vi "Avvia pompa.vi"(0 "Valvole avvio":T1, 1 "Tipo motore pompa":enum16{"Monofase", "Trifase"}(ring), 5 "Indici valvole linea":i16[](array[numeric]), 7 "V F rpm avvio":T2, 9 "V F rpm prova":T2, 12 "Reset avvio":bool) -> (6 "Fine Avvio":bool=TRUE, 10 "stato":string)   [LabVIEW 2019]
uses:
  Global_All_Data.vi
  cDAQ_PLC Folder/cDAQ/DO List.ctl
  cDAQ_PLC Folder/cDAQ/SET SINGLE DO.ctl
  cDAQ_PLC Folder/cDAQ/SET ARRAY DO.ctl
  cDAQ_PLC Folder/cDAQ/AO List.ctl
  cDAQ_PLC Folder/cDAQ/SET SINGLE AO.ctl
  SubVI ELETTROTEST60A Folder/Elettrotest60A/Global_bypass_ResMeter.vi
  Global SCELTA LINEA.vi
  Gestione Inverter/STATUS VACON.vi
panel:
  out "Stato":string
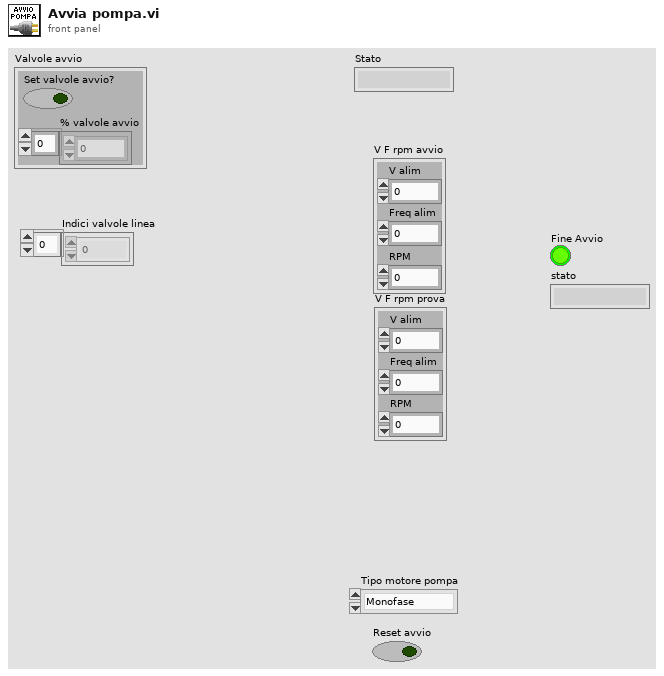
[diagram p1: front panel]
types:
  T1 = cluster{"Set valvole avvio?":bool, "% valvole avvio":dbl[]}
  T2 = cluster{"V alim":dbl, "Freq alim":dbl, "RPM":dbl}
  T3 = enum16{"Alimentazione diretta", "Variac/inverter", "Pompa trascinata"}
  T4 = enum16{"LINEA 135A BYPASS TRASFO", "LINEA 15A BYPASS TRASFO", "LINEA 135A TRASFO 400V", "LINEA 135A TRASFO 500V", "LINEA 15A TRASFO 400V", "LINEA 15A TRASFO 500V", "LINEA 2", "NESSUNA LINEA SELEZIONATA"}
  T5 = cluster{"Array of elements":cluster{"String":string, "variant":variant}[], "Single element":cluster{"String":string, "variant":variant}, "enque at\nopposite end (F)":bool, "no replications (F)":bool}
  T6 = typedef "SET ARRAY DO.ctl" = T7[]
  T7 = typedef "SET SINGLE DO.ctl" = cluster{"DO":T8, "Value":bool}
  T8 = typedef "DO List.ctl" = enum16{"OFF: ALL DO", "*ABILITA freno 1", "*ABILITA freno 2", "*ABILITA freno 3", "*START freno 1", "*START freno 2", "*START freno 3", "*STOP freno 1", "*STOP freno 3", "*STOP freno 2", "*Senso rot freno 1", "*Senso rot freno 2", "*Senso rot freno 3", "*Ctrl velocità freno 1", "*Ctrl velocità freno 2", "*Ctrl velocità freno 3", "*Ctrl coppia freno 1", "*Ctrl coppia freno 2", "*Ctrl coppia freno 3", "*ABILITA alimentatore 1", "*ABILITA alimentatore 2", "*ABILITA alimentatore 3", "*ABILITA alimentatore 4", "*START alimentatore 1", "*START alimentatore 2", "*START alimentatore 3", "*START alimentatore 4", "*STOP alimentatore 1", "*STOP alimentatore 2", "*STOP alimentatore 3", "*STOP alimentatore 4", "SENSO ROT alimentatore 1", "SENSO ROT alimentatore 2", "Abilita LEM 1000A", "Abilita LEM 300A", "Abilita sensori EXT WT", "B1 Seleziona linea 1", "B1 Seleziona linea 2", "B1 Seleziona linea 3", "B1 Seleziona linea 4", "B1 Seleziona linea 5", "B2 Seleziona linea 1", "B2 Seleziona linea 2", "B2 Seleziona linea 3", "B2 Seleziona linea 4", "B2 Seleziona linea 5", "*Reset allarmi", "*Start potenza AC", "*Stop potenza AC", "*Start potenza DC", "*Stop potenza DC", "*Start potenza DC eccit", "*Stop pontenza DC eccit", "Bypass res meter", "2nd canale res meter", "Enable res meter", "*Abilit teler ramo WT", "*Abil teler ramo princ Resit", "*Abil teler ramo 1 Resist", "*Abil teler ramo 2 Resist", "*Abil teler ramo 3 Resist", "*Abil cortocirc avvolgim", "*Controllo torsiometro B1", "*Controllo Torsiom B2", "*Scala torsiometro B1", "*Scala torsiometro B2", "*Collaudo in corso", "*Allarme presente", "Abilitazione elettroserratura", "Exit", "*Abilita collaudo", "*Abilita potenza trifase", "*Abilita potenza monofase", "*Abilita potenza DC", "*Abilita potenza DC eccit", "*Disabilita teleruttori potenza", "Set teleruttori prova a freddo", "Prova a freddo monofase", "Watchdog", "Forza DO PLC 3", "Forza DO PLC 2", "Forza DO PLC 1", "Forza DO cDAQ", "Scala 2000(T) 200(F) res meter", "Seleziona banco 1", "Seleziona banco 2", "Comando azionam in blocco", "Comando azionam reset", "Sensibilità freno 16 32 nm", "Reset Allarmi", "Carico res - Ramo 1", "Carico res - Ramo 2", "Carico res - Ramo 3", "Carico res - Ramo 4", "Carico res - Ramo 5", "Carico res - Ramo 6", "Carico res - Ramo 7", "Carico res - Ramo 8", "Carico res - Ramo 9", "Carico res - Ramo 10", "Carico res - Ramo 11", "Carico res - Start ventilatore", "Carico res - Stop ventilatore", "Abilita potenza solo freno", "Abilita AFE + freno trasc", "Abilita potenza carico resistivo", "Chiudi potenza AFE", "Apri potenza AFE", "Start AFE", "Config Banco2 TDE", "Misura diretto WT", "Ripristina centralina protezioni", "Abilita Scrittura Dati Keb"}
  T9 = typedef "SET SINGLE AO.ctl" = cluster{"AO":T10, "Value":dbl}
  T10 = typedef "AO List.ctl" = enum16{"OFF: ALL AO", "Valvola prop 1", "Valvola prop 2", "Valvola prop 3", "Valvola prop 4", "Valvola prop 5", "Valvola prop 6", "Vavlola prop 7", "Valvola prop 8", "Valvola prop 9", "Valvola prop 10", "Rif vel motore trasc 1", "Rif vel motore trasc 2", "Rif vel motore trasc 3", "Rif vel motore pompa boost 1", "Rif vel motore pompa boost 2", "Rif vel motore pompa boost 3", "Rif Vout", "Rif Freq out", "FORZA AO", "Exit"}
  T11 = typedef "Cluster MISURE.ctl" = cluster{"MISURE NM":T12, "MISURE ALL":T13}
  T12 = typedef "MISURE NM.ctl" = cluster{"Banco":string, "Anno":string, "Numero":string, "Ntabella":string, "Misura":string, "Tipo Prova":string, "ProgressivoAcq":string, "Descrizione":string, "Data_ora":string, "t. acq [h:m:s]":string, "t. acq [min]":string, "t. acq [s]":string, "n [rpm]":string, "f [Hz]":string, "U1[V]":string, "U2 [V]":string, "U3 [V]":string, "U123_media [V]":string, "I1[A]":string, "I2[A]":string, "I3[A]":string, "I123_media [A]*I":string, "I_123_sbil [%]":string, "Ulin[V]":string, "Uc [V]":string, "Uaux [V]":string, "Ilin[A]*I":string, "Imar[A]":string, "Iaux[A]":string, "Uarm[V]":string, "Uecc[V]":string, "Iarm[A]*I":string, "Iecc[A]":string, "pf":string, "P1 [W]":string, "P1 [kW]":string, "Q [VAR]":string, "Q [kVAR]":string, "S [VA]":string, "S [kVA]":string, "P1arm[W]":string, "P1ecc[W]":string, "Parm[kW]":string, "P1ecc[kW]":string, "Cond[uF]":string, "P1_linea_6fili[W]":string, "P1_linea_6fili[kW]":string, "eta_gr_6fili [%]":string, "eta_inverter_6fili [%]":string, "pf_linea_6fili":string, "U4 [V]":string, "U5 [V]":string, "U6 [V]":string, "U456_media [V]":string, "I4 [A]":string, "I5 [A]":string, "I6 [A]":string, "I456_media [A]":string, "C [Nm]*C":string, "Cric [Nm]":string, "Cric\\Cnom":string, "Iric[A]":string, "Iric\\Inom":string, "P2_mecc [W]":string, "P2_mecc [kW]":string, "eta motore [%]":string, "Scorr[%]":string, "Tamb[°C]":string, "R1[ohm]":string, "R2[ohm]":string, "R3[ohm]":string, "Rmedia[ohm]":string, "DT_R1[°C]":string, "DT_R2[°C]":string, "DT_R3[°C]":string, "DT_media[°C]":string, "R_marcia[ohm]":string, "R_aux[ohm]":string, "DT_marcia[°C]":string, "DT_aux[°C]":string, "R_Arm[ohm]":string, "R_Ecc[ohm]":string, "DT_Arm[°C]":string, "DT_Ecc[°C]":string, "TambFreddo[°C]":string, "R1_freddo[ohm]":string, "R2_freddo[ohm]":string, "R3_freddo[ohm]":string, "Rmedia_freddo[ohm]":string, "R_Marcia_freddo[ohm]":string, "R_Aux_freddo[ohm]":string, "R_Arm_freddo[ohm]":string, "R_Ecc_freddo[ohm]":string, "TC1 [°C]":string, "TC2 [°C]":string, "TC3 [°C]":string, "TC4 [°C]":string, "TC5 [°C]":string, "TC6 [°C]":string, "TC7 [°C]":string, "TC8 [°C]":string, "PT1000_1[°C]":string, "PT1000_2[°C]":string, "PT1000_3[°C]":string, "Vdc eccitatrice[V]":string, "Idc eccitatrice[A]":string, "Vdc rotore[V]":string, "Idc rotore[A]":string, "Vac rotore[V]":string, "Iac rotore[V]":string, "V dinamo[V]":string, "Portata Q":string, "Pressione H":string, "U1'[V]":string, "U2'[V]":string, "U3'[V]":string, "I1'[A]":string, "I2'[A]":string, "I3'[A]":string, "U''R-N":string, "U''S-N":string, "U'' T-N":string, "U''R-S":string, "U''R-T":string, "U''S-T":string, "I1''[A]":string, "I2''[A]":string, "I3''[A]":string, "F''[Hz]":string, "P''[kW]":string, "CosFi''":string, "PT1000_4[°C]":string, "Scorta 3":string}
  T13 = typedef "Cluster misure ALL.ctl" = cluster{"Cluster READ NI":T14, "MISURE WT":T17, "Resistenze Resistomat":T18, "INTERFACCIA":T19, "FREDDO resistomat":cluster{"Res Ch1":dbl, "Res Ch2":dbl, "tAMB":dbl, "Res Ch3":dbl}, "STATO PLC 1":T24, "Res Ch2":dbl, "Res Ch2 2":dbl, "FREDDO res meter":cluster{"Res Ch1":dbl, "Res Ch2":dbl, "tAMB":dbl, "Res Ch3":dbl}, "Resistenze Res Meter":T18, "READ SINUS PENTA":T28, "STATO PLC 2":T29, "STATO PLC 3":T33, "DCREG":T37}
  T14 = typedef "Cluster NI.ctl" = cluster{"AI (0-10V)":cluster{"AI 0":dbl, "AI 1":dbl, "AI 2":dbl, "AI 3":dbl, "AI 4":dbl, "AI 5":dbl, "AI 6":dbl, "AI 7":dbl, "AI 8":dbl, "AI 9":dbl, "AI 10":dbl, "AI 11":dbl, "AI 12":dbl, "AI 13":dbl, "AI 14":dbl, "AI 15":dbl, "AI 16":dbl, "AI 17":dbl, "AI 18":dbl, "AI 19":dbl, "AI 20":dbl, "AI 21":dbl, "AI 22":dbl, "AI 23":dbl, "AI 24":dbl, "AI 25":dbl, "AI 26":dbl, "AI 27":dbl, "AI 28":dbl, "AI 29":dbl, "AI 30":dbl, "AI 31":dbl}, "StatoAO_Cdaq[0-10V]":cluster{"AO 1":dbl, "AO 2":dbl, "AO 3":dbl, "AO 4":dbl}, "Contatori [rpm]":cluster{"RPM 1":dbl, "RPM 2":dbl}, "StatoAO_Cdaq [4-20mA]":T15, "StatoDO_Cdaq":T16, "DI":cluster{"Scorta 0":bool, "Scorta 1":bool, "Scorta 2":bool, "Scorta 3":bool, "Scorta 4":bool, "Scorta 5":bool, "Scorta 6":bool, "Scorta 7":bool, "Scorta 8":bool, "Scorta 9":bool, "Scorta 10":bool, "Scorta 11":bool, "Scorta 12":bool, "Scorta 13":bool, "Scorta 14":bool, "Scorta 15":bool, "Scorta 16":bool, "Scorta 17":bool, "Scorta 18":bool, "Scorta 19":bool, "Scorta 20":bool, "Scorta 21":bool, "Scorta 22":bool, "Scorta 23":bool, "Scorta 24":bool, "Scorta 25":bool, "Scorta 26":bool, "Scorta 27":bool, "Scorta 28":bool, "Scorta 29":bool, "Scorta 30":bool, "Scorta 31":bool}, "AI (4-20mA)":cluster{"AI 0":dbl, "AI 1":dbl, "AI 2":dbl, "AI 3":dbl, "AI 4":dbl, "AI 5":dbl, "AI 6":dbl, "AI 7":dbl, "AI 8":dbl, "AI 9":dbl, "AI 10":dbl, "AI 11":dbl, "AI 12":dbl, "AI 13":dbl, "AI 14":dbl, "AI 15":dbl}, "TC [°C]":cluster{"tc 1":dbl, "tc 2":dbl, "tc 3":dbl, "tc 4":dbl}}
  T15 = typedef "StatoAO_cdaq.ctl" = cluster{"Cdaq_AO [0-10V] 0":dbl, "Cdaq_AO [0-10V] 1":dbl, "Cdaq_AO [0-10V] 2":dbl, "Cdaq_AO [0-10V] 3":dbl, "Cdaq_AO [4-20mA] 0":dbl, "Cdaq_AO [4-20mA] 1":dbl, "Cdaq_AO [4-20mA] 2":dbl, "Cdaq_AO [4-20mA] 3":dbl, "Cdaq_AO [4-20mA] 4":dbl, "Cdaq_AO [4-20mA] 5":dbl, "Cdaq_AO [4-20mA] 6":dbl, "Cdaq_AO [4-20mA] 7":dbl}
  T16 = typedef "statoDO_Cdaq.ctl" = cluster{"Scorta 0":bool, "Scorta 1":bool, "Scorta 2":bool, "Scorta 3":bool, "Scorta 4":bool, "Scorta 5":bool, "Scorta 6":bool, "Scorta 7":bool, "Scorta 8":bool, "Scorta 9":bool, "Scorta 10":bool, "Scorta 11":bool, "Scorta 12":bool, "Scorta 13":bool, "Scorta 14":bool, "Scorta 15":bool, "Scorta 16":bool, "Scorta 17":bool, "Scorta 18":bool, "Scorta 19":bool, "Scorta 20":bool, "Scorta 21":bool, "Scorta 22":bool, "Scorta 23":bool, "Scorta 24":bool, "Scorta 25":bool, "Scorta 26":bool, "Scorta 27":bool, "Scorta 28":bool, "Scorta 29":bool, "Scorta 30":bool, "Scorta 31":bool}
  T17 = typedef "MISURE WT.ctl" = cluster{"URMS 1":dbl, "IRMS 1":dbl, "P 1":dbl, "S 1":dbl, "Q 1":dbl, "LAMBDA 1":dbl, "PHI 1":dbl, "F U 1":dbl, "F I 1":dbl, "NONE 1":dbl, "URMS 2":dbl, "IRMS 2":dbl, "P 2":dbl, "S 2":dbl, "Q 2":dbl, "LAMBDA 2":dbl, "PHI 2":dbl, "F U 2":dbl, "F I 2":dbl, "NONE 2":dbl, "URMS 3":dbl, "IRMS 3":dbl, "P 3":dbl, "S 3":dbl, "Q 3":dbl, "LAMBDA 3":dbl, "PHI 3":dbl, "F U 3":dbl, "F I 3":dbl, "NONE 3":dbl, "URMS 4":dbl, "IRMS 4":dbl, "P 4":dbl, "S 4":dbl, "Q 4":dbl, "LAMBDA 4":dbl, "PHI 4":dbl, "F U 4":dbl, "F I 4":dbl, "NONE 4":dbl, "URMS 5":dbl, "IRMS 5":dbl, "P 5":dbl, "S 5":dbl, "Q 5":dbl, "LAMBDA 5":dbl, "PHI 5":dbl, "F U 5":dbl, "F I 5":dbl, "NONE 5":dbl, "URMS 6":dbl, "IRMS 6":dbl, "P 6":dbl, "S 6":dbl, "Q 6":dbl, "LAMBDA 6":dbl, "PHI 6":dbl, "F U 6":dbl, "F I 6":dbl, "NONE 6":dbl, "URMS SIGMA":dbl, "IRMS SIGMA":dbl, "P SIGMA":dbl, "S SIGMA":dbl, "Q SIGMA":dbl, "LAMBDA SIGMA":dbl, "PHI SIGMA":dbl, "F U SIGMA":dbl, "F I SIGMA":dbl, "NONE 7":dbl, "URMS SIGMB":dbl, "IRMS SIGMB":dbl, "P SIGMB":dbl, "S SIGMB":dbl, "Q SIGMB":dbl, "LAMBDA SIGMB":dbl, "PHI SIGMB":dbl, "F U SIGMB":dbl, "F I SIGMB":dbl, "NONE 8":dbl, "URMS SIGMC":dbl, "IRMS SIGMC":dbl, "P SIGMC":dbl, "S SIGMC":dbl, "Q SIGMC":dbl, "LAMBDA SIGMC":dbl, "PHI SIGMC":dbl, "F U SIGMC":dbl, "F I SIGMC":dbl, "NONE 9":dbl, "SPEED":dbl, "TORQUE[Nm]":dbl, "Pmecc[kW]":dbl}
  T18 = typedef "ClusterRes.ctl" = cluster{"Res Ch1":dbl, "Res Ch2":dbl, "Res Ch3":dbl, "Tamb":dbl}
  T19 = typedef "INTERFACCIA.ctl" = cluster{"AI":cluster{"Portate":T20[], "Pressioni":T20[], "Coppie[Nm]":T20[], "Valvole prop %":T20[], "RPM":T20[], "Livelli":T20[], "Temperature":T20[], "Riferimenti %":T20[], "TENSIONI":T20[], "CORRENTI":T20[]}, "DI (logici)":cluster{"Start da pulsantiera":bool, "Stop da pulsantiera":bool, "Reset da pulsantiera":bool, "Sistema OK":bool, "Collaudo abilitato":bool, "Potenza trifase abilitata":bool, "Potenza monofase abilitata":bool, "Potenza DC abilitata":bool, "Potenza DC ECC abilitata":bool, "Start alimentazione AC":bool, "Start alimentazione DC":bool, "Start DC eccitazione":bool, "Teleruttore WT abilitato":bool, "Teleruttore Resistomat abilitato":bool, "Teleruttore corto fasi":bool, "Ramo 1 resistomat":bool, "Ramo 2 resistomat":bool, "Ramo 3 resistomat":bool, "B1 Scelta linea elettrica 1":bool, "B1 Scelta linea elettrica 2":bool, "B1 Scelta linea elettrica 3":bool, "B1 Scelta linea elettrica 4":bool, "B1 Scelta linea elettrica 5":bool, "B2 Scelta linea elettrica 1":bool, "B2 Scelta linea elettrica 2":bool, "B2 Scelta linea elettrica 3":bool, "B2 Scelta linea elettrica 4":bool, "B2 Scelta linea elettrica 5":bool, "Rotore bloccato 1":bool, "Rotore bloccato 2":bool, "FRENO 1 abilitato":bool, "FRENO 1 run":bool, "FRENO 1 senso rotaz":bool, "FRENO 1 ctrl velocità":bool, "FRENO 2 abilitato":bool, "FRENO 2 run":bool, "FRENO 2 senso rotaz":bool, "FRENO 2 ctrl velocità":bool, "ALIM 1 abilitato":bool, "ALIM 1 run":bool, "ALIM 2 abilitato":bool, "ALIM 2 run":bool, "ALIM 3 abilitato":bool, "ALIM 3 run":bool, "FRENO 1 ctrl coppia":bool, "FRENO 2 ctrl coppia":bool, "FRENO 3 ctrl coppia":bool, "DI (logici) aggiuntivi impianto":cluster{"Solo freno abilitato":bool, "Carico resistivo abilitato":bool, "AFE+freno abilitato":bool, "Protezioni chiuse":bool, "Start potenza AFE":bool, "AFE in marcia":bool}, "Misura corrente diretta WT":bool, "Misura corrente sens ext":bool, "Sens ext abilitati":bool}, "AO non scalati":T22, "AO scalati":T22, "DO (logici)":T23}
  T20 = typedef "ClusterMisura_e_Unità_INPUT.ctl" = cluster{"Misura":dbl, "UM":T21, "Descrizione":string}
  T21 = typedef "UnitàMisura.ctl" = enum16{"V", "mA", "Bar", "RPM", "m3/s", "m3/min", "m3/h", "l/s", "l/min", "in3/min", "ft3/min", "gpm", "igpm", "igph", "%", "°C", "m", "Nm", "A"}
  T22 = typedef "Lista AO sistema.ctl" = cluster{"FRENO1 rif vel":dbl, "FRENO1 rif Coppia":dbl, "FRENO2 rif vel":dbl, "FRENO2 rif Coppia":dbl, "ALIM1 rif V":dbl, "ALIM1 rif F":dbl, "ALIM2 rif V":dbl, "ALIM2 rif F":dbl, "ALIM3 rif V":dbl, "ALIM3 rif F":dbl, "Fnom keb":dbl, "Rpm nom keb":dbl, "Pnom keb":dbl, "Inom keb":dbl, "Vnom keb":dbl, "Rpm max keb":dbl, "Tempo rampa keb":dbl, "Tipo Mot keb":dbl}
  T23 = typedef "DOinterfaccia.ctl" = cluster{"Scelta banco 1":bool, "Scelta banco 2":bool, "Scelta banco 3":bool, "FRENO 1 abilita":bool, "FRENO 1 start":bool, "FRENO 1 senso rotaz":bool, "FRENO 1 ctrl velocità":bool, "FRENO 2 abilita":bool, "FRENO 2 start":bool, "FRENO 2 senso rotaz":bool, "FRENO 2 ctrl velocità":bool, "ALIM 1 abilita":bool, "ALIM 1 start":bool, "ALIM 2 abilita":bool, "ALIM 2 start":bool, "ALIM 3 abilita":bool, "ALIM 3 start":bool, "Abilita linea trifase":bool, "Abilita linea monofase":bool, "Abilita linea dc":bool, "Abilita linea dc eccit":bool, "B1 Linea elettrica 1":bool, "B1 Linea elettrica 2":bool, "B1 Linea elettrica 3":bool, "B1 Linea elettrica 4":bool, "B1 Linea elettrica 5":bool, "B2 Linea elettrica 1":bool, "B2 Linea elettrica 2":bool, "B2 Linea elettrica 3":bool, "B2 Linea elettrica 4":bool, "B2 Linea elettrica 5":bool, "Start potenza AC":bool, "Stop pontenza AC":bool, "Start potenza DC":bool, "Stop potenza DC":bool, "Start potenza eccitaz":bool, "Stop potenza eccitaz":bool, "Reset allarmi":bool, "watchdog":bool, "Scala torsiometro B1":bool, "Controllo torsiom B1":bool, "Scala torsiometro B2":bool, "Controllo torsiom B2":bool, "Teleruttore WT abilita":bool, "Teleruttore Resistomat abilita":bool, "Teleruttore corto fasi":bool, "Ramo 1 resistomat":bool, "Ramo 2 resistomat":bool, "Ramo 3 resistomat":bool, "Collaudo in corso":bool, "Allarme presente":bool, "Enable Res Meter":bool, "Bypass Res Meter":bool, "2nd canale Res Meter":bool, "Scala 200/2000 res meter":bool, "Taratura res meter":bool, "FRENO 1 ctrl coppia":bool, "FRENO 2 ctrl coppia":bool, "FRENO 3 ctrl coppia":bool, "Aggiuntivi impianto":cluster{"Senso rotazione alim 1":bool, "Senso rotazione alim 2":bool}, "ALIM 1 stop":bool, "ALIM 2 stop":bool, "ALIM 3 stop":bool, "FRENO 1 stop":bool, "FRENO 2 stop":bool, "FRENO 3 stop":bool, "B1 configurazione freno B":bool, "B2 configurazione freno B":bool, "Abilita scrittura KEB":bool}
  T24 = typedef "STATO PLC 1.ctl" = cluster{"USCITE PLC":T25, "Stato DI_PLC":cluster{"Sistema OK":bool, "Rotore bloccato":bool, "Scorta 1":bool, "Prova diretto inverter":bool, "Prova con filtro LC":bool, "Teleruttore WT abilitato":bool, "Alim sinus penta abilitato":bool, "Alim sinus penta in marcia":bool, "Freno abilitato":bool, "Freno in marcia":bool, "Senso rotazione freno":bool, "Potenza abilitata":bool, "Scorta 3":bool, "Scorta 4":bool, "scorta 5":bool, "scorta 6":bool}, "AI plc":cluster{"Allarmi 1":dbl, "Allarmi 2":dbl, "Scorta 1":dbl, "Scorta 2":dbl, "RPM mot prova":dbl, "I mot prova":dbl, "RPM freno":dbl, "I freno":dbl, "Scorta 3":dbl, "Scorta 4":dbl}}
  T25 = typedef "Uscite PLC 1.ctl" = cluster{"AO (real) 2":cluster{"SCORTA 1":dbl, "SCORTA 2":dbl, "SCORTA 3":dbl, "SCORTA 4":dbl, "SCORTA 5":dbl, "SCORTA 6":dbl, "SCORTA 7":dbl, "SCORTA 8":dbl}, "statoAO_PLC out":T26, "DO (bit)":T27}
  T26 = typedef "statoAO_plc_1.ctl" = cluster{"Rif Lim coppia freno [%]":dbl, "Rif rpm freno [%]":dbl, "Rif coppia freno [%]":dbl, "Rif V alimentatore [%]":dbl, "Rif F alimentatore [%]":dbl}
  T27 = typedef "StatoDO_PLC_1.ctl" = cluster{"Scelta banco 1":bool, "Set dati motore freno 2":bool, "Diretto inverter":bool, "Filtro LC":bool, "Marcia ALIM (1s)":bool, "Marcia FRENO (1s)":bool, "Stop AFE (1s)":bool, "Stop freno (1s)":bool, "Reset allarmi":bool, "Watchdog":bool, "Senso rotazione":bool, "Abilita collaudo (1s)":bool, "Disabilita collaudo (1s)":bool, "Abilitazione ALIM":bool, "Abilitazione FRENO":bool, "Teleruttore WT":bool, "Senso rot motore prova":bool, "Scorta 7":bool, "Scorta 8":bool, "Scorta 9":bool, "Scorta 10":bool, "Scorta 11":bool, "Scorta 12":bool, "Scorta 13":bool}
  T28 = typedef "Parametri inverter letti.ctl" = cluster{"Menù Misure motore (M000-M030)":cluster{"Rif vel a regime (int)":u16, "Rif vel a regime (dec)":u16, "Rif vel dopo rampe (int)":u16, "Rif vel dopo rampe (dec)":u16, "RPM motore (int)":u16, "RPM motore (dec)":u16, "FREQout inverter":u16, "Rif coppia a regime(Nm)":u16, "Richiesta di coppia (Nm)":u16, "Coppia generata dal motore(Nm)":u16, "Rif coppia a regime(%)":u16, "Richiesta di coppia (%)":u16, "Coppia generata dal motore(%)":u16, "Coppia max richiesta prima delle rampe(Nm)":u16, "Coppia max richiesta dopo le rampe(Nm)":u16, "Limite di velocità prima delle rampe":u16, "Limite di velocità dopo le rampe":u16, "Coppia max richiesta prima delle rampe(%)":u16, "Coppia max richiesta dopo le rampe(%)":u16, "Rif di flusso":u16, "Corrente di uscita":u16, "Capacità termica del motore":u16, "Tensione di uscita":u16, "Potenza di uscita":u16, "Energia consumata (LSword)":u16, "Energia consumata (MSword)":u16, "Tensione bus DC":u16, "Tensione di rete":u16}, "Menù regolatore PID (M018-M024)":cluster{"Rif PID a regime(%)":u16, "Rif pid dopo rampe(%)":u16, "Retroazione del pid(%)":u16, "Errore del pid(%)":u16, "uscita del pid(%)":u16, "Rif del pid dopo le rampe":u16, "Retroazione del pid":u16}, "Menù ingressi digitali (M031-M036)":cluster{"Ingressi digitali ritardati":u16, "Ingressi digitali istantanei":u16, "Moresettiera comando loc":u16, "Morsett comando da seriale":u16, "Morsett comando bus di campo":u16, "Ing dig ausiliari da morsettiera":u16, "Ing dig ausiliari da seriale":u16}, "Menù riferimenti (M037-M051)":cluster{"Rif analog est REF":u16, "Rif analog est AIN1":u16, "Rif analog est AIN2":u16, "Rif analog est XAIN4":u16, "Rif analog est XAIN5":u16, "Rif velocità da seriale(int)":u16, "Rif velocità bus di campo(int)":u16, "Rif coppia da seriale":u16, "Rif coppia bus di campo":u16, "Rif del PID da seriale":u16, "Rif del PID da bus di campo":u16, "Retroazione del PID da seriale":u16, "Retroazione del PIDda bus di campo":u16, "Rif da encoder":u16, "Rif in frequenza":u16, "Rif velocità da seriale(dec)":u16, "Rif velocità bus di campo(dec)":u16}, "Menù rampe (P009-P033)":cluster{"Tempo di dec rampa di vel 1":u16, "Tempo di acc rampa di vel 2":u16, "Tempo di dec rampa di vel 2":u16, "Tempo di acc rampa di vel 1":u16, "Unità di mis tempi rampe vel 1/2":u16, "Tempo di acc rampa di vel 3":u16, "Tempo di dec rampa di vel 3":u16, "Tempo di acc rampa di vel 4":u16, "Tempo di dec rampa di vel 4":u16, "Unità di mis tempi rampe vel 3/4":u16, "Selettore arrottondam rampe":u16, "Tempo di arrotond iniz rampa acc":u16, "Tempo di arrotond finale rampa acc":u16, "Tempo di arrotond iniz rampa dec":u16, "Tempo di rampa di salita rif coppia":u16, "Tempo di rampa di discesa rif coppia":u16, "Unità di misura rampa coppia":u16, "Tempo rampa acc marcia jog":u16, "Tempo rampa dec marcia jog":u16, "Reset acc ai cambi pendenza":u16, "rampa di acc in fire mode":u16, "rampa di dec in fire mode":u16, "Tempo di arrotond finale rampa dec":u16}, "Menù controllo motore(C008-C128)":cluster{"Numero motori configurati":u16, "Tipo algoritmo di controllo Mot1":u16, "Tipo rif Mot1":u16, "Tensione nominale rete":u16, "Retroaz di vel da encoder Mot1":u16, "Tipo curva V/f Mot1":u16, "Rotazione delle fasi Mot1":u16, "Freq nominale del motore Mot1":u16, "RPM nominali del motore Mot1":u16, "Potenza nominale del motore Mot1":u16, "Corrente nominale del motore Mot1":u16, "Tensione nominale del motore mot1":u16, "Potenza a vuoto del motore Mot1":u16, "Corrente a vuoto del motore Mot1":u16, "Resistenza statorica del motore Mot1":u16, "Induttanza di dispersione Mot1":u16, "Induttanza mutua motore":u16, "Costante di tempo rotorica":u16, "Costante di tempo filtro pb":u16, "Velocità minima motore":u16, "Velocità massima motore":u16}, "Menù configurazione PID":cluster{"Selezione riferimento n.1":u16, "Selezione retroazione n.1":u16, "Modalità di fuzionamento PID":u16, "Termine derivativo calcolato su err o mis":u16, "Proporz moltiplica deriv e integrale":u16, "Azione del PID":u16}, "ID":dbl, "Menù uscite digitali":cluster{"MDO4 Inverter pronto":u16}, "Fcarrier":cluster{"Fcarrier Min (Hz)":u16, "Fcarrier Max (Hz)":u16}, "stato inverter M089":dbl, "Riferimenti":cluster{"Rif tensione":u16, "Rif velocità":u16}, "Comunicazione":bool, "Modalità stop":dbl}
  T29 = typedef "STATO PLC 2.ctl" = cluster{"USCITE PLC":T30, "Stato DI_PLC":cluster{"Sistema ok":bool, "Relè Resistomat abilitato":bool, "scorta d":bool, "scorta c":bool, "scorta b":bool, "scorta a":bool, "scorta 1":bool, "scorta 2":bool, "scorta 3":bool, "scorta 4":bool, "Scorta 5":bool, "Scorta 6":bool, "Scorta 7":bool, "Scorta 8":bool, "Scorta 9":bool, "Scorta 10":bool}, "AI plc":cluster{"Allarmi 1":dbl, "Allarmi 2":dbl, "TC 1":dbl, "TC 2":dbl, "TC 3":dbl, "TC 4":dbl, "TC 5":dbl, "TC 6":dbl, "TC 7":dbl, "TC 8":dbl, "PT1000 1":dbl, "PT1000 2":dbl, "PT1000 3":dbl, "PT1000 4":dbl}}
  T30 = typedef "Uscite PLC 2.ctl" = cluster{"AO (real) 2":cluster{"SCORTA 1":dbl, "SCORTA 2":dbl, "SCORTA 3":dbl, "SCORTA 4":dbl, "SCORTA 5":dbl, "SCORTA 6":dbl, "SCORTA 7":dbl, "SCORTA 8":dbl}, "statoAO_PLC out":T31, "DO (bit)":T32}
  T31 = typedef "statoAO_plc_2.ctl" = cluster{"Condensatori":dbl, "Scorta 1":dbl, "Scorta 2":dbl}
  T32 = typedef "StatoDO_PLC_2.ctl" = cluster{"Scala Torsiometro":bool, "Ctrl torsiometro":bool, "Relè misura resistomat":bool, "Watchdog":bool, "Misura res ramo 1":bool, "Misura res ramo 2":bool, "Misura res ramo 3":bool, "Scelta banco 2":bool, "Reset allarmi":bool, "Reset centraline":bool, "Scorta 2":bool, "Scorta 3":bool, "Scorta 4":bool, "Scorta 5":bool, "Scorta 6":bool, "Scorta 7":bool}
  T33 = typedef "STATO PLC 3.ctl" = cluster{"USCITE PLC":T34, "Stato DI_PLC":cluster{"Sistema OK":bool, "Rotore bloccato":bool, "Filtro LC":bool, "Bypass Filtro LC":bool, "Scelta Trasformatore":bool, "Scelta Bypass trasformatore":bool, "Teleruttore wt abilitato":bool, "Alimentatore abilitato":bool, "Alimentatore in marcia":bool, "Freno abilitato":bool, "Freno in marcia":bool, "Freno senso di rotazione":bool, "Potenza abilitata":bool, "Alimentatore in allarme":bool, "Freno in allarme":bool, "Conferma dati KEB":bool, "Scorta 4":bool, "Scorta 5":bool, "Scorta 6":bool}, "AI plc":cluster{"Allarmi 1":dbl, "Allarmi 2":dbl, "RPM motore prova":dbl, "Corrente motore prova":dbl, "RPM freno":dbl, "Corrente freno":dbl, "Tipo motore keb":dbl, "I nom keb":dbl, "RPM nom keb":dbl, "V nom keb":dbl, "F nom keb":dbl, "T rampa keb":dbl, "scorta":dbl, "Scorta 2":dbl}}
  T34 = typedef "Uscite PLC 3.ctl" = cluster{"AO (real) 2":cluster{"SCORTA 1":dbl, "SCORTA 2":dbl, "SCORTA 3":dbl, "SCORTA 4":dbl, "SCORTA 5":dbl, "SCORTA 6":dbl, "SCORTA 7":dbl, "SCORTA 8":dbl}, "statoAO_PLC out":T35, "DO (bit)":T36}
  T35 = typedef "statoAO_plc_3.ctl" = cluster{"Rif limitazione coppia freno":dbl, "Rif velocità freno":dbl, "Rif coppia freno (predisp.)":dbl, "Rif velocità alimentatore":dbl, "Scorta":dbl, "Tipo Motore  keb":dbl, "I nom keb":dbl, "RPM nom keb":dbl, "V nom keb":dbl, "F nom keb":dbl, "t rampa keb":dbl, "scorta":dbl, "Scorta 2":dbl}
  T36 = typedef "StatoDO_PLC_3.ctl" = cluster{"Scelta banco 2":bool, "Abilita Scrittura Dati Keb":bool, "Filtro LC":bool, "Bypass filtro LC":bool, "Trasformatore":bool, "Bypass trasformatore":bool, "Marcia alimentatore (1s)":bool, "Marcia freno (1s)":bool, "Stop alimentatore (1s)":bool, "Stop freno (1s)":bool, "Reset allarmi":bool, "Watchdog":bool, "Freno senso di rotazione":bool, "Abilita pontenza (1s)":bool, "Disabilita potenza (1s)":bool, "Abilita alimentatore":bool, "Abilita freno":bool, "Teleruttore wt":bool, "Senso rot mot prova":bool, "Scorta":bool, "Scorta":bool, "Blocco elettroserrature":bool, "Scorta 6":bool, "Scorta 7":bool}
  T37 = typedef "Parametri DCREG letti.ctl" = cluster{"Parametri di misura":cluster{"M000":dbl, "M001":dbl, "M002":dbl, "M003":dbl, "M004":dbl, "M005":dbl, "M006":dbl, "M007":dbl, "M008":dbl, "M009":dbl, "M010":dbl, "M011":dbl, "M012":dbl, "M013":dbl, "M014":dbl, "M015":dbl, "M016":dbl, "M017":dbl, "M018":dbl, "M019":dbl, "M020":dbl, "M021":dbl, "M022":dbl, "M023":dbl, "M024":dbl, "M025":dbl, "M026":dbl, "M027":dbl, "M028":dbl, "M029":dbl, "M030":dbl, "M031":dbl}, "Parametri di programmazione":cluster{"P000":dbl, "P001":dbl, "P002":dbl, "P003":dbl, "P004":dbl, "P005":dbl, "P006":dbl, "P010":dbl, "P011":dbl, "P012":dbl, "P013":dbl, "P014":dbl, "P015":dbl, "P016":dbl, "P030":dbl, "P031":dbl, "P032":dbl, "P033":dbl, "P034":dbl, "P035":dbl, "P036":dbl, "P037":dbl, "P038":dbl, "P039":dbl, "P040":dbl, "P050":dbl, "P051":dbl, "P052":dbl, "P053":dbl, "P054":dbl, "P055":dbl, "P056":dbl, "P057":dbl, "P058":dbl, "P059":dbl, "P060":dbl, "P061":dbl, "P062":dbl, "P070":dbl, "P071":dbl, "P073":dbl, "P074":dbl, "P076":dbl, "P077":dbl, "P079":dbl, "P080":dbl, "P082":dbl, "P083":dbl, "P084":dbl, "P085":dbl, "P086":dbl, "P087":dbl, "P088":dbl, "P100":dbl, "P101":dbl, "P102":dbl, "P103":dbl, "P104":dbl, "P110":dbl, "P111":dbl, "P120":dbl, "P121":dbl, "P122":dbl, "P123":dbl, "P124":dbl, "P125":dbl, "P126":dbl, "P127":dbl, "P128":dbl, "P129":dbl, "P130":dbl, "P131":dbl, "P132":dbl, "P133":dbl, "P134":dbl, "P150":dbl, "P151":dbl, "P152":dbl, "P153":dbl, "P154":dbl, "P155":dbl, "P156":dbl, "P157":dbl, "P158":dbl, "P170":dbl, "P171":dbl, "P172":dbl, "P173":dbl, "P174":dbl, "P175":dbl, "P176":dbl, "P177":dbl, "P178":dbl, "P179":dbl, "P180":dbl, "P181":dbl, "P182":dbl, "P183":dbl, "P184":dbl, "P185":dbl, "P186":dbl, "P187":dbl, "P188":dbl, "P189":dbl, "P190":dbl, "P191":dbl, "P192":dbl, "P193":dbl, "P194":dbl, "P195":dbl, "P196":dbl, "P197":dbl, "P198":dbl, "P199":dbl, "P211":dbl, "P212":dbl, "P213":dbl, "P214":dbl, "P215":dbl, "P216":dbl, "P217":dbl, "P221":dbl, "P222":dbl, "P223":dbl, "P224":dbl, "P230":dbl, "P231":dbl, "P240":dbl, "P250":dbl, "P251":dbl}, "Parametri di configurazione":cluster{"C000":dbl, "C001":dbl, "C002":dbl, "C010":dbl, "C011":dbl, "C012":dbl, "C014":dbl, "C015":dbl, "C016":dbl, "C017":dbl, "C018":dbl, "C030":dbl, "C050":dbl, "C051":dbl, "C052":dbl, "C060":dbl, "C061":dbl, "C062":dbl, "C063":dbl, "C070":dbl, "C072":dbl, "C074":dbl, "C090":dbl, "C091":dbl, "C092":dbl, "C093":dbl, "C094":dbl, "C100":dbl, "C101":dbl, "C102":dbl, "C103":dbl, "C105":dbl, "C106":dbl, "C107":dbl, "C108":dbl, "C110":dbl, "C111":dbl, "C112":dbl, "C120":dbl, "C121":dbl, "C122":dbl, "C130":dbl, "C131":dbl, "C132":dbl, "C133":dbl, "C134":dbl, "C135":dbl, "C141":dbl, "C142":dbl, "C143":dbl, "C150":dbl, "C151":dbl, "C153":dbl, "C154":dbl, "C155":dbl, "C156":dbl, "C157":dbl, "C158":dbl, "C159":dbl, "C160":dbl, "C161":dbl, "C162":dbl, "C163":dbl, "C164":dbl, "C165":dbl, "C170":dbl}, "Codice allarme":dbl, "Comunicazione":bool}
  T38 = cluster{"READY":bool, "RUN":bool, "CW(F) CCW(T)":bool, "FAULTED":bool, "WARNING":bool, "REF. FREQ. REACHED":bool, "MOTOR RUNNING AT 0 SPEED":bool, "FLUX READY":bool, "TC SPEED NOT ACTIVE":bool, "ENCODER DIRECTION CCW":bool, "UV FAST STOP NOT ACTIVE":bool, "NOT USED":bool}
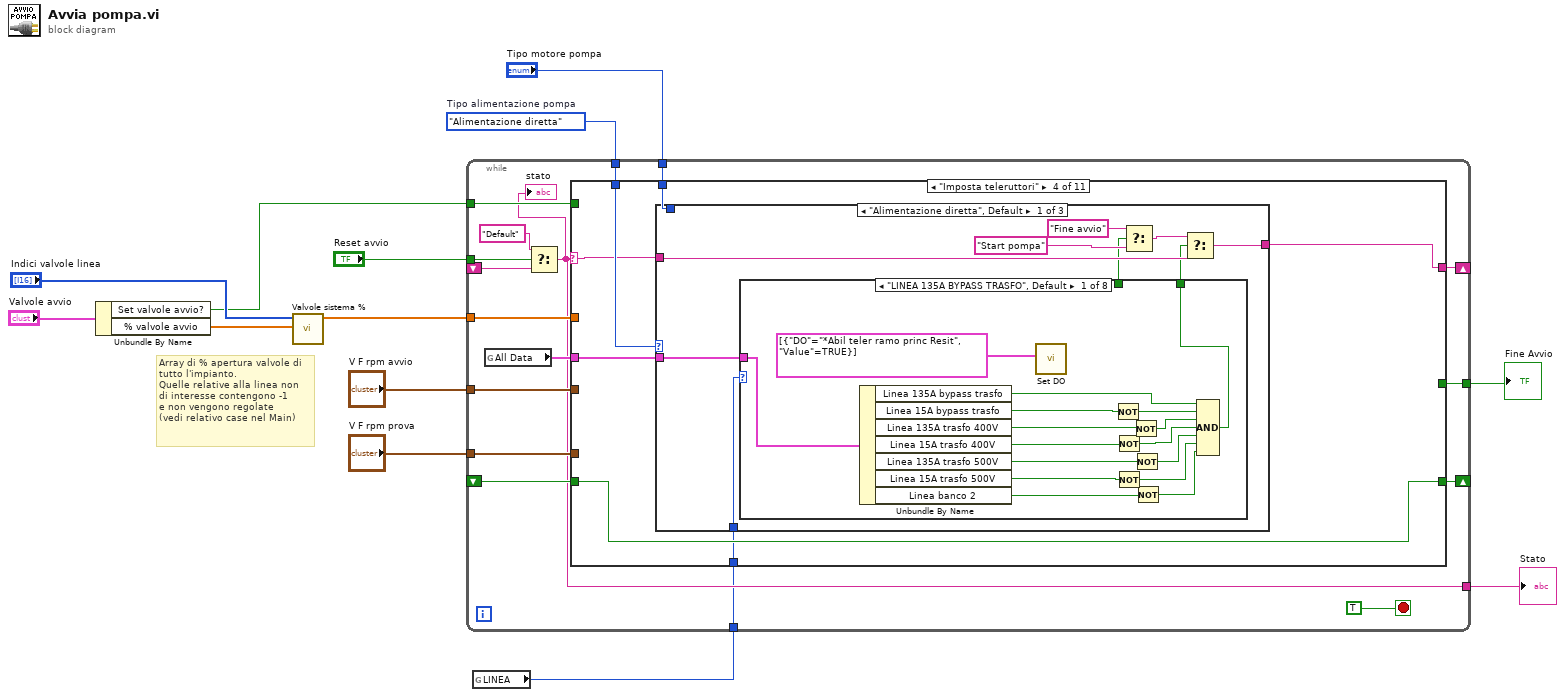
[diagram p0: block diagram]
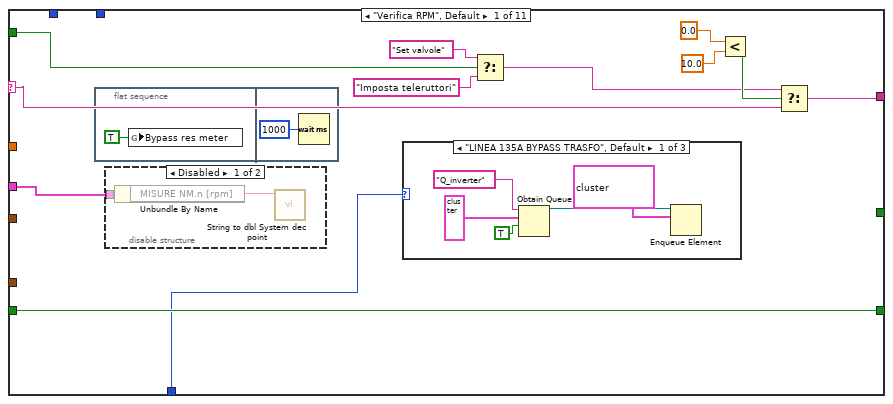
[diagram p2: hidden frame]
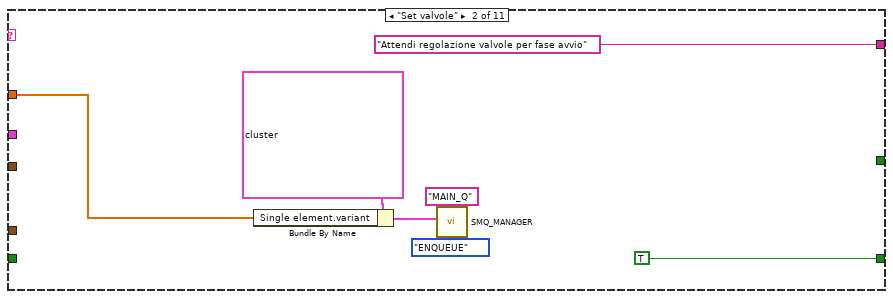
[diagram p6: hidden frame]
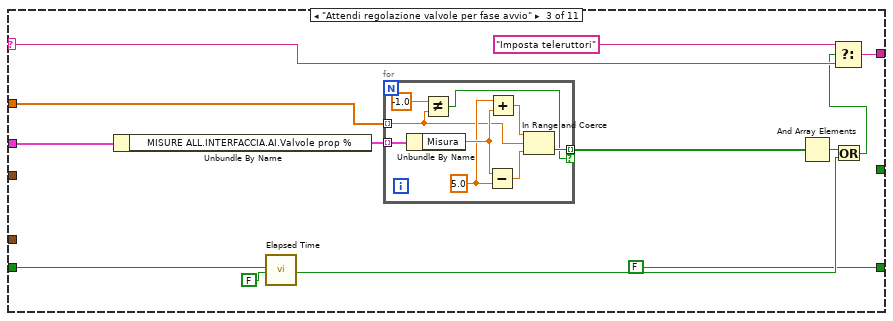
[diagram p7: hidden frame]
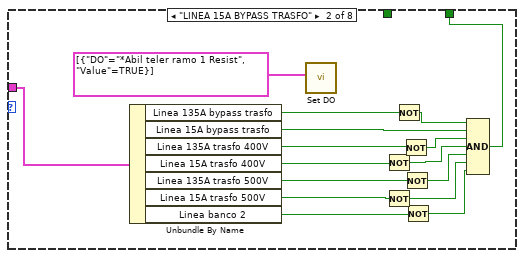
[diagram p8: hidden frame]
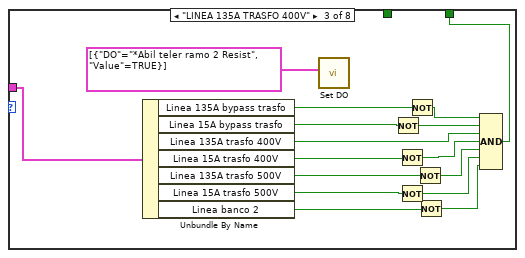
[diagram p9: hidden frame]
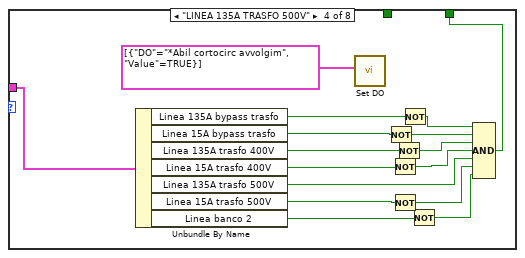
[diagram p10: hidden frame]
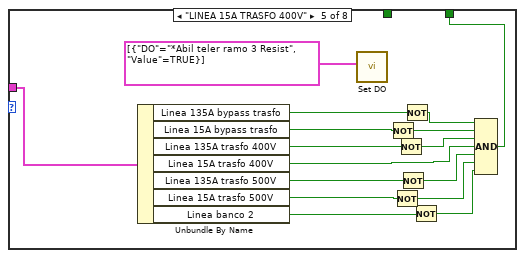
[diagram p11: hidden frame]
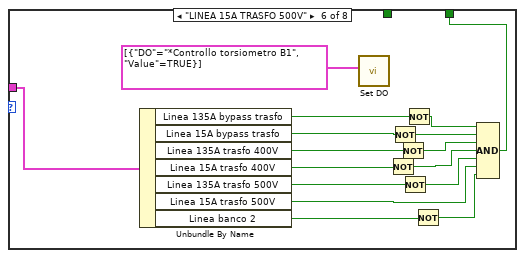
[diagram p12: hidden frame]
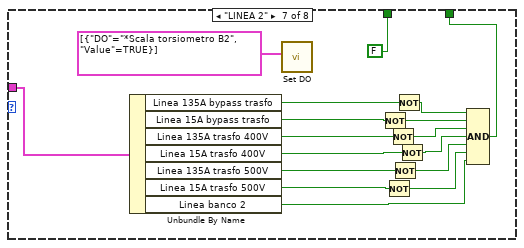
[diagram p13: hidden frame]
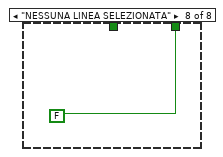
[diagram p14: hidden frame]
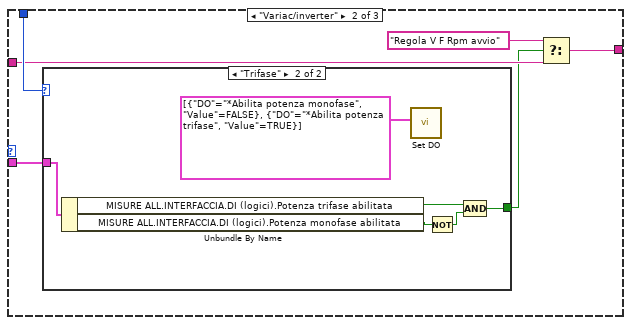
[diagram p15: hidden frame]
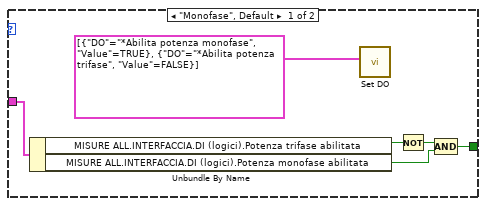
[diagram p16: hidden frame]
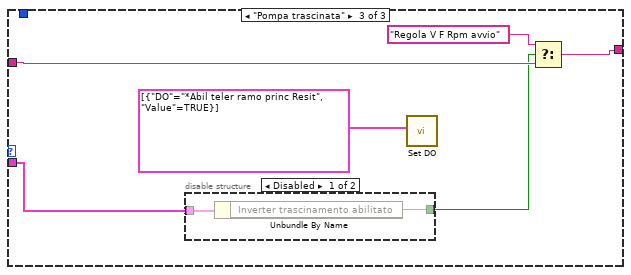
[diagram p17: hidden frame]
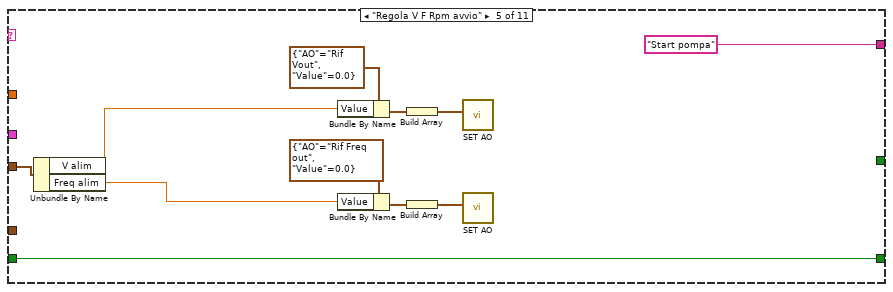
[diagram p19: hidden frame]
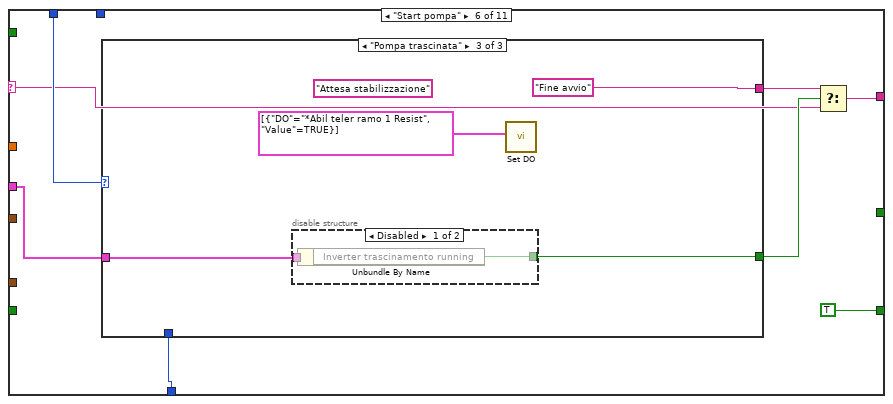
[diagram p20: hidden frame]
diagram:
  w12 = T3."Alimentazione diretta"  # Tipo alimentazione pompa
  # "Array di % apertura valvole di\ntutto l'impianto.\nQuelle relative alla linea non\ndi interesse contengono -1\ne non vengono regolate\n(vedi relativo case nel Main)"
  n1 = Unbundle By Name("Valvole avvio") -> ("Set valvole avvio?"=w3:bool, "% valvole avvio"=w7:dbl[])
  n2 = call "Valvole sistema %.vi"("% valvole linea"=w7, "Indici valvole linea"="Indici valvole linea") -> ("Array Valvole sistema out %"=w4:dbl[])  [unwired: 9 in]
  n3 = global read "Global SCELTA LINEA.vi" "LINEA"() -> (w1:T4)
  n4 = while {
    shift-right: [w29] -> _
    shift-left: _ -> [w28]
    tunnel: "Reset avvio" -> [w26]
    tunnel: w12 -> [w24]
    tunnel: w3 -> [w23]
    tunnel: w4 -> [w22]
    shift-right: [w21] -> _
    shift-left: _ -> [w20]
    tunnel: "Tipo motore pompa" -> [w19]
    tunnel: "V F rpm avvio" -> [w18]
    tunnel: "V F rpm prova" -> [w17]
    tunnel: [w16] -> w8
    tunnel: [w15] -> w2
    tunnel: w1 -> [w14]
    stop <- TRUE stop-if-true
    n5 = global read "Global_All_Data.vi" "All Data"() -> (w25:T11)
    n6 = Select(t="Default", s=w26, f=w28) -> (s? t:f=w15:string)
    "stato" <- w15
    n7 = case shown="\"Imposta teleruttori\"" w15 {
      selector: w15 -> [w39 _ w70 w83 _ w252 w287 _ _ w324 _]
      tunnel: [w38 "Attendi regolazione valvole per fase avvio" ("t") w69 w82 "Start pompa" ("t") w251 w286 w296 "Attesa stabilizzazione 2" ("t") w323 _] -> w29
      tunnel: w25 -> [w42 _ w68 w84 _ w254 _ _ _ _ _]
      tunnel: w24 -> [_ _ _ w87 _ w255 _ w294 _ _ _]
      tunnel: w23 -> [w35 _ _ _ _ _ _ _ _ _ _]
      tunnel: w22 -> [_ w55 w66 _ _ _ _ _ _ _ _]
      tunnel: [w33 TRUE ("Auto Reset") FALSE ("Auto Reset") w86 w237 TRUE ("Auto Reset") FALSE ("Auto Reset") w299 TRUE ("Auto Reset") FALSE ("Auto Reset") w346] -> w21
      tunnel: w20 -> [w33 _ w59 w86 w237 _ w290 w299 _ w319 w346]
      tunnel: w19 -> [_ _ _ w85 _ _ _ _ _ _ _]
      tunnel: w18 -> [_ _ _ _ w244 _ _ _ _ _ _]
      tunnel: w17 -> [_ _ _ _ _ _ _ _ w308 _ _]
      tunnel: [_ _ _ _ _ _ _ _ _ _ TRUE] -> w16
      tunnel: w14 -> [w31 _ _ w81 _ w248 _ _ _ w321 _]
      frame "Verifica RPM", Default {
        n8 = flat-sequence {
          frame #0 {
            n9 = global write "Global_bypass_ResMeter.vi" "Bypass res meter"(TRUE ("Bypass res meter")) -> ()
          }
          frame #1 {
            n10 = Wait (ms)(milliseconds to wait=u32 1000) -> ()  [unwired: 1 out]
          }
        }
        n11 = disable-structure shown="Disabled" {
          disable-tunnel: w42 -> [w51 _]
          frame Disabled {
            n12 = Unbundle By Name(w51) -> ("MISURE NM.n [rpm]"=w50:string)
            n13 = call "String to dbl System dec point.vi"("n [rpm]"=w50) -> ()  [unwired: 10 in, 1 out]
          }
          frame Enabled {
          }
        }
        n14 = case shown="\"LINEA 135A BYPASS TRASFO\", Default" w31 {
          frame "LINEA 135A BYPASS TRASFO", Default {
            n15 = Obtain Queue(name (unnamed)="Q_inverter" ("name"), element data type=cluster{"DATA":variant, "status":string} {"DATA"=variant, "status"=""} ("output cluster"), create if not found? (T)=TRUE) -> (queue out=w45:refnum<queue>)  [unwired: 2 in, 2 out]
            n16 = Enqueue Element(queue=w45, element=cluster{"DATA":variant, "status":string} {"DATA"=variant, "status"="Reset allarmi"}) -> ()  [unwired: 2 in, 3 out]
          }
          frame "LINEA 2" {
          }
          frame "NESSUNA LINEA SELEZIONATA" {
          }
        }
        n17 = Select(t="Set valvole", s=w35, f="Imposta teleruttori" ("t")) -> (s? t:f=w34:string)
        n18 = Less?(x=0.0, y=10.0) -> (x < y?=w40:bool)
        n19 = Select(t=w34, s=w40, f=w39) -> (s? t:f=w38:string)
      }
      frame "Set valvole" {
        n20 = Bundle By Name(cluster=T5 {"Array of elements"=[], "Single element"={"String"="COMANDI VALVOLE PROP", "variant"=variant}, "enque at\nopposite end (F)"=FALSE, "no replications (F)"=FALSE} ("Enqueue cluster"), "Single element.variant"=w55) -> (w56:T5)
        n21 = call <userlib>:"SMQ_MANAGER.vi"("Function"=enum16{"INITIALIZE", "ENQUEUE", "STOP ALL"}."ENQUEUE", "Queue name"="MAIN_Q", "Enqueue cluster"=w56) -> ()  [unwired: 8 in, 1 out]
      }
      frame "Attendi regolazione valvole per fase avvio" {
        n22 = Unbundle By Name(w68) -> ("MISURE ALL.INTERFACCIA.AI.Valvole prop %"=w67:T20[])
        n23 = call "Elapsed Time"("Reset"=w59, "Auto Reset"=FALSE) -> ("Time has Elapsed"=w63:bool)  [unwired: 10 in, 7 out]
        n24 = for {
          tunnel: w67 -> [w80] mode=indexing
          tunnel: w66 -> [w74] mode=indexing
          tunnel: [w75] -> w65 mode=indexing if=w72
          w76 = 5.0 ("y")
          n25 = Unbundle By Name(w80) -> ("Misura"=w77:dbl)
          n26 = Not Equal?(x=-1.0, y=w74) -> (x != y?=w72:bool)
          n27 = Subtract(x=w77, y=w76) -> (x-y=w79:dbl)
          n28 = Add(x=w76, y=w77) -> (x+y=w78:dbl)
          n29 = In Range and Coerce(upper limit=w78, x=w74, lower limit=w79) -> (In Range?=w75:bool)  [unwired: 1 out]
        }
        n30 = And Array Elements(Boolean array=w65) -> (logical AND=w64:bool)
        n31 = Or(x=w64, y=w63) -> (x .or. y?=w62:bool)
        n32 = Select(t="Imposta teleruttori", s=w62, f=w70) -> (s? t:f=w69:string)
      }
      frame "Imposta teleruttori" {
        n33 = case shown="\"Alimentazione diretta\", Default" w87 {
          tunnel: w85 -> [_ w215 _]
          tunnel: w84 -> [w93 w214 w233]
          tunnel: w83 -> [w96 w213 w232]
          tunnel: [w95 w211 w229] -> w82
          tunnel: w81 -> [w94 _ _]
          frame "Alimentazione diretta", Default {
            n34 = case shown="\"LINEA 135A BYPASS TRASFO\", Default" w94 {
              tunnel: w93 -> [w111 w116 w132 w145 w164 w180 w197 _]
              tunnel: [w97 w113 w129 w146 w161 w177 w194 FALSE] -> w92
              tunnel: [_ _ _ _ _ _ FALSE _] -> w88
              frame "LINEA 135A BYPASS TRASFO", Default {
                n35 = Unbundle By Name(w111) -> ("Linea 135A bypass trasfo"=w103:bool, "Linea 15A bypass trasfo"=w110:bool, "Linea 135A trasfo 400V"=w108:bool, "Linea 15A trasfo 400V"=w107:bool, "Linea 135A trasfo 500V"=w106:bool, "Linea 15A trasfo 500V"=w105:bool, "Linea banco 2"=w104:bool)
                n36 = call "Set DO.vi"("Cluster SET DO"=T6 [{"DO"=enum."*Abil teler ramo princ Resit", "Value"=TRUE}]) -> ()  [unwired: 10 in, 1 out]
                n37 = Not(x=w110) -> (.not. x?=w109:bool)
                n38 = Not(x=w107) -> (.not. x?=w101:bool)
                n39 = Not(x=w105) -> (.not. x?=w99:bool)
                n40 = Not(x=w108) -> (.not. x?=w102:bool)
                n41 = Not(x=w106) -> (.not. x?=w100:bool)
                n42 = Not(x=w104) -> (.not. x?=w98:bool)
                n43 = Compound Arithmetic op=AND(w103, w109, w102, w101, w100, w99, w98) -> (w97:bool)
              }
              frame "LINEA 15A BYPASS TRASFO" {
                n44 = Unbundle By Name(w116) -> ("Linea 135A bypass trasfo"=w122:bool, "Linea 15A bypass trasfo"=w114:bool, "Linea 135A trasfo 400V"=w127:bool, "Linea 15A trasfo 400V"=w126:bool, "Linea 135A trasfo 500V"=w125:bool, "Linea 15A trasfo 500V"=w124:bool, "Linea banco 2"=w123:bool)
                n45 = call "Set DO.vi"("Cluster SET DO"=T6 [{"DO"=enum."*Abil teler ramo 1 Resist", "Value"=TRUE}]) -> ()  [unwired: 10 in, 1 out]
                n46 = Not(x=w126) -> (.not. x?=w120:bool)
                n47 = Not(x=w124) -> (.not. x?=w118:bool)
                n48 = Not(x=w122) -> (.not. x?=w115:bool)
                n49 = Not(x=w127) -> (.not. x?=w121:bool)
                n50 = Not(x=w125) -> (.not. x?=w119:bool)
                n51 = Not(x=w123) -> (.not. x?=w117:bool)
                n52 = Compound Arithmetic op=AND(w115, w114, w121, w120, w119, w118, w117) -> (w113:bool)
              }
              frame "LINEA 135A TRASFO 400V" {
                n53 = Unbundle By Name(w132) -> ("Linea 135A bypass trasfo"=w139:bool, "Linea 15A bypass trasfo"=w133:bool, "Linea 135A trasfo 400V"=w130:bool, "Linea 15A trasfo 400V"=w143:bool, "Linea 135A trasfo 500V"=w142:bool, "Linea 15A trasfo 500V"=w141:bool, "Linea banco 2"=w140:bool)
                n54 = call "Set DO.vi"("Cluster SET DO"=T6 [{"DO"=enum."*Abil teler ramo 2 Resist", "Value"=TRUE}]) -> ()  [unwired: 10 in, 1 out]
                n55 = Not(x=w133) -> (.not. x?=w131:bool)
                n56 = Not(x=w143) -> (.not. x?=w138:bool)
                n57 = Not(x=w141) -> (.not. x?=w136:bool)
                n58 = Not(x=w139) -> (.not. x?=w134:bool)
                n59 = Not(x=w142) -> (.not. x?=w137:bool)
                n60 = Not(x=w140) -> (.not. x?=w135:bool)
                n61 = Compound Arithmetic op=AND(w134, w131, w130, w138, w137, w136, w135) -> (w129:bool)
              }
              frame "LINEA 135A TRASFO 500V" {
                n62 = Unbundle By Name(w145) -> ("Linea 135A bypass trasfo"=w157:bool, "Linea 15A bypass trasfo"=w152:bool, "Linea 135A trasfo 400V"=w150:bool, "Linea 15A trasfo 400V"=w160:bool, "Linea 135A trasfo 500V"=w147:bool, "Linea 15A trasfo 500V"=w159:bool, "Linea banco 2"=w158:bool)
                n63 = call "Set DO.vi"("Cluster SET DO"=T6 [{"DO"=enum."*Abil cortocirc avvolgim", "Value"=TRUE}]) -> ()  [unwired: 10 in, 1 out]
                n64 = Not(x=w152) -> (.not. x?=w151:bool)
                n65 = Not(x=w160) -> (.not. x?=w156:bool)
                n66 = Not(x=w159) -> (.not. x?=w155:bool)
                n67 = Not(x=w150) -> (.not. x?=w148:bool)
                n68 = Not(x=w157) -> (.not. x?=w153:bool)
                n69 = Not(x=w158) -> (.not. x?=w154:bool)
                n70 = Compound Arithmetic op=AND(w153, w151, w148, w156, w147, w155, w154) -> (w146:bool)
              }
              frame "LINEA 15A TRASFO 400V" {
                n71 = Unbundle By Name(w164) -> ("Linea 135A bypass trasfo"=w174:bool, "Linea 15A bypass trasfo"=w170:bool, "Linea 135A trasfo 400V"=w168:bool, "Linea 15A trasfo 400V"=w162:bool, "Linea 135A trasfo 500V"=w165:bool, "Linea 15A trasfo 500V"=w176:bool, "Linea banco 2"=w175:bool)
                n72 = call "Set DO.vi"("Cluster SET DO"=T6 [{"DO"=enum."*Abil teler ramo 3 Resist", "Value"=TRUE}]) -> ()  [unwired: 10 in, 1 out]
                n73 = Not(x=w170) -> (.not. x?=w169:bool)
                n74 = Not(x=w176) -> (.not. x?=w173:bool)
                n75 = Not(x=w168) -> (.not. x?=w166:bool)
                n76 = Not(x=w165) -> (.not. x?=w163:bool)
                n77 = Not(x=w174) -> (.not. x?=w171:bool)
                n78 = Not(x=w175) -> (.not. x?=w172:bool)
                n79 = Compound Arithmetic op=AND(w171, w169, w166, w162, w163, w173, w172) -> (w161:bool)
              }
              frame "LINEA 15A TRASFO 500V" {
                n80 = Unbundle By Name(w180) -> ("Linea 135A bypass trasfo"=w191:bool, "Linea 15A bypass trasfo"=w188:bool, "Linea 135A trasfo 400V"=w186:bool, "Linea 15A trasfo 400V"=w181:bool, "Linea 135A trasfo 500V"=w183:bool, "Linea 15A trasfo 500V"=w178:bool, "Linea banco 2"=w192:bool)
                n81 = call "Set DO.vi"("Cluster SET DO"=T6 [{"DO"=enum."*Controllo torsiometro B1", "Value"=TRUE}]) -> ()  [unwired: 10 in, 1 out]
                n82 = Not(x=w181) -> (.not. x?=w179:bool)
                n83 = Not(x=w188) -> (.not. x?=w187:bool)
                n84 = Not(x=w186) -> (.not. x?=w184:bool)
                n85 = Not(x=w183) -> (.not. x?=w182:bool)
                n86 = Not(x=w191) -> (.not. x?=w189:bool)
                n87 = Not(x=w192) -> (.not. x?=w190:bool)
                n88 = Compound Arithmetic op=AND(w189, w187, w184, w179, w182, w178, w190) -> (w177:bool)
              }
              frame "LINEA 2" {
                n89 = Unbundle By Name(w197) -> ("Linea 135A bypass trasfo"=w208:bool, "Linea 15A bypass trasfo"=w205:bool, "Linea 135A trasfo 400V"=w203:bool, "Linea 15A trasfo 400V"=w198:bool, "Linea 135A trasfo 500V"=w200:bool, "Linea 15A trasfo 500V"=w209:bool, "Linea banco 2"=w195:bool)
                n90 = call "Set DO.vi"("Cluster SET DO"=T6 [{"DO"=enum."*Scala torsiometro B2", "Value"=TRUE}]) -> ()  [unwired: 10 in, 1 out]
                n91 = Not(x=w205) -> (.not. x?=w204:bool)
                n92 = Not(x=w209) -> (.not. x?=w207:bool)
                n93 = Not(x=w203) -> (.not. x?=w201:bool)
                n94 = Not(x=w200) -> (.not. x?=w199:bool)
                n95 = Not(x=w208) -> (.not. x?=w206:bool)
                n96 = Not(x=w198) -> (.not. x?=w196:bool)
                n97 = Compound Arithmetic op=AND(w206, w204, w201, w196, w199, w207, w195) -> (w194:bool)
              }
              frame "NESSUNA LINEA SELEZIONATA" {
              }
            }
            n98 = Select(t="Fine avvio", s=w88, f="Start pompa" ("t")) -> (s? t:f=w90:string)
            n99 = Select(t=w90, s=w92, f=w96) -> (s? t:f=w95:string)
          }
          frame "Variac/inverter" {
            n100 = case shown="\"Trifase\"" w215 {
              tunnel: w214 -> [w221 w227]
              tunnel: [w219 w223] -> w212
              frame "Monofase", Default {
                n101 = Unbundle By Name(w221) -> ("MISURE ALL.INTERFACCIA.DI (logici).Potenza trifase abilitata"=w220:bool, "MISURE ALL.INTERFACCIA.DI (logici).Potenza monofase abilitata"=w218:bool)
                n102 = call "Set DO.vi"("Cluster SET DO"=T6 [{"DO"=enum."*Abilita potenza monofase", "Value"=TRUE}, {"DO"=enum."*Abilita potenza trifase", "Value"=FALSE}]) -> ()  [unwired: 10 in, 1 out]
                n103 = Not(x=w220) -> (.not. x?=w217:bool)
                n104 = Compound Arithmetic op=AND(w217, w218) -> (w219:bool)
              }
              frame "Trifase" {
                n105 = Unbundle By Name(w227) -> ("MISURE ALL.INTERFACCIA.DI (logici).Potenza trifase abilitata"=w224:bool, "MISURE ALL.INTERFACCIA.DI (logici).Potenza monofase abilitata"=w226:bool)
                n106 = call "Set DO.vi"("Cluster SET DO"=T6 [{"DO"=enum."*Abilita potenza monofase", "Value"=FALSE}, {"DO"=enum."*Abilita potenza trifase", "Value"=TRUE}]) -> ()  [unwired: 10 in, 1 out]
                n107 = Not(x=w226) -> (.not. x?=w225:bool)
                n108 = Compound Arithmetic op=AND(w224, w225) -> (w223:bool)
              }
            }
            n109 = Select(t="Regola V F Rpm avvio", s=w212, f=w213) -> (s? t:f=w211:string)
          }
          frame "Pompa trascinata" {
            n110 = disable-structure shown="Disabled" {
              disable-tunnel: w233 -> [w236 _]
              disable-tunnel: [w235 _] -> w231
              frame Disabled {
                n111 = Unbundle By Name(w236) -> ("Inverter trascinamento abilitato"=w235:bool)
              }
              frame Enabled {
              }
            }
            n112 = call "Set DO.vi"("Cluster SET DO"=T6 [{"DO"=enum."*Abil teler ramo princ Resit", "Value"=TRUE}]) -> ()  [unwired: 10 in, 1 out]
            n113 = Select(t="Regola V F Rpm avvio", s=w231, f=w232) -> (s? t:f=w229:string)
          }
        }
      }
      frame "Regola V F Rpm avvio" {
        n114 = Unbundle By Name(w244) -> ("V alim"=w243:dbl, "Freq alim"=w239:dbl)
        n115 = Bundle By Name(cluster=T9 {"AO"=enum."Rif Vout", "Value"=0.0} ("Cluster SET AO"), "Value"=w243) -> (w246:T9)
        n116 = Bundle By Name(cluster=T9 {"AO"=enum."Rif Freq out", "Value"=0.0} ("Cluster SET AO"), "Value"=w239) -> (w241:T9)
        n117 = Build Array(w246) -> (w245:T9[])
        n118 = Build Array(w241) -> (w242:T9[])
        n119 = call "SET AO.vi"("Cluster SET AO"=w245) -> ()  [unwired: 10 in, 1 out]
        n120 = call "SET AO.vi"("Cluster SET AO"=w242) -> ()  [unwired: 10 in, 1 out]
      }
      frame "Start pompa" {
        n121 = case shown="\"Pompa trascinata\"" w255 {
          tunnel: w254 -> [w262 w277 w281]
          tunnel: [w258 w276 w280] -> w253
          tunnel: ["Attesa stabilizzazione 2" ("t") "Attesa stabilizzazione" ("t") "Fine avvio" ("t")] -> w250
          tunnel: w248 -> [w257 _ _]
          frame "Alimentazione diretta", Default {
            n122 = flat-sequence {
              frame #0 {
                n123 = call "Set DO.vi"("Cluster SET DO"=T6 [{"DO"=enum."OFF: ALL DO", "Value"=TRUE}]) -> ()  [unwired: 10 in, 1 out]
              }
              frame #1 {
                n124 = Wait (ms)(milliseconds to wait=u32 1000) -> ()  [unwired: 1 out]
              }
              frame #2 {
                n125 = call "Set DO.vi"("Cluster SET DO"=T6 [{"DO"=enum."OFF: ALL DO", "Value"=FALSE}]) -> ()  [unwired: 10 in, 1 out]
              }
            }
            n126 = Unbundle By Name(w262) -> ("MISURE ALL.INTERFACCIA.DI (logici).Potenza DC abilitata"=w259:bool)
            n127 = case shown="\"LINEA 135A BYPASS TRASFO\", Default" w257 {
              tunnel: [w263 w264 w265 w266 w267 w268 w269 w271] -> w260
              tunnel: TRUE -> [w263 w264 w265 w266 w267 w268 _ w271]
              frame "LINEA 135A BYPASS TRASFO", Default {
              }
              frame "LINEA 15A BYPASS TRASFO" {
              }
              frame "LINEA 135A TRASFO 400V" {
              }
              frame "LINEA 135A TRASFO 500V" {
              }
              frame "LINEA 15A TRASFO 400V" {
              }
              frame "LINEA 15A TRASFO 500V" {
              }
              frame "LINEA 2" {
                n128 = global read "STATUS VACON.vi" "STATUS VACON"() -> (w270:T38)
                n129 = Unbundle By Name(w270) -> ("READY"=w269:bool)
              }
              frame "NESSUNA LINEA SELEZIONATA" {
              }
            }
            n130 = And(x=w260, y=w259) -> (x .and. y?=w258:bool)
          }
          frame "Variac/inverter" {
            n131 = Unbundle By Name(w277) -> ("MISURE ALL.INTERFACCIA.DI (logici).Potenza DC abilitata"=w276:bool)
            n132 = call "Set DO.vi"("Cluster SET DO"=T6 [{"DO"=enum."OFF: ALL DO", "Value"=TRUE}]) -> ()  [unwired: 10 in, 1 out]
          }
          frame "Pompa trascinata" {
            (unwired) "Attesa stabilizzazione" ("t")
            n133 = disable-structure shown="Disabled" {
              disable-tunnel: w281 -> [w284 _]
              disable-tunnel: [w283 _] -> w280
              frame Disabled {
                n134 = Unbundle By Name(w284) -> ("Inverter trascinamento running"=w283:bool)
              }
              frame Enabled {
              }
            }
            n135 = call "Set DO.vi"("Cluster SET DO"=T6 [{"DO"=enum."*Abil teler ramo 1 Resist", "Value"=TRUE}]) -> ()  [unwired: 10 in, 1 out]
          }
        }
        n136 = Select(t=w250, s=w253, f=w252) -> (s? t:f=w251:string)
      }
      frame "Attesa stabilizzazione" {
        n137 = call "Elapsed Time2"("Time Target (s)"=3.0, "Reset"=w290, "Auto Reset"=FALSE) -> ("Time has Elapsed"=w288:bool)  [unwired: 9 in, 7 out]
        n138 = Select(t="Fine avvio", s=w288, f=w287) -> (s? t:f=w286:string)
      }
      frame "Abilita wattmetro" {
        w295 = T3."Alimentazione diretta"  # Tipo alimentazione pompa
        n139 = flat-sequence {
          frame #0 {
            n140 = call "Set DO.vi"("Cluster SET DO"=T6 [{"DO"=enum."OFF: ALL DO", "Value"=TRUE}]) -> ()  [unwired: 10 in, 1 out]
          }
          frame #1 {
            n141 = Wait (ms)(milliseconds to wait=u32 500) -> ()  [unwired: 1 out]
          }
          frame #2 {
            n142 = call "Set DO.vi"("Cluster SET DO"=T6 [{"DO"=enum."OFF: ALL DO", "Value"=FALSE}]) -> ()  [unwired: 10 in, 1 out]
          }
        }
        n143 = Equal?(x=w294, y=w295) -> (x = y?=w293:bool)
        n144 = Select(t="Fine avvio", s=w293, f="Regola V F Rpm prova" ("t")) -> (s? t:f=w296:string)
      }
      frame "Regola V F Rpm prova" {
        n145 = Unbundle By Name(w308) -> ("V alim"=w307:dbl, "Freq alim"=w306:dbl, "RPM"=w305:dbl)
        n146 = Bundle By Name(cluster=T9 {"AO"=enum."Rif vel motore trasc 1", "Value"=0.0} ("Cluster SET AO"), "Value"=w305) -> (w316:T9)
        n147 = Bundle By Name(cluster=T9 {"AO"=enum."Rif Vout", "Value"=0.0} ("Cluster SET AO"), "Value"=w307) -> (w313:T9)
        n148 = Bundle By Name(cluster=T9 {"AO"=enum."Rif Freq out", "Value"=0.0} ("Cluster SET AO"), "Value"=w306) -> (w310:T9)
        n149 = Build Array(w316) -> (w315:T9[])
        n150 = Build Array(w313) -> (w312:T9[])
        n151 = Build Array(w310) -> (w311:T9[])
        n152 = call "SET AO.vi"("Cluster SET AO"=w315) -> ()  [unwired: 10 in, 1 out]
        n153 = call "SET AO.vi"("Cluster SET AO"=w312) -> ()  [unwired: 10 in, 1 out]
        n154 = call "SET AO.vi"("Cluster SET AO"=w311) -> ()  [unwired: 10 in, 1 out]
      }
      frame "Attesa stabilizzazione 2" {
        n155 = call "Elapsed Time3"("Time Target (s)"=3.0, "Reset"=w319, "Auto Reset"=FALSE) -> ("Time has Elapsed"=w318:bool)  [unwired: 9 in, 7 out]
        n156 = case shown="\"LINEA 2\"" w321 {
          tunnel: [w328 w329 w330 w331 w332 w333 w334 w343] -> w320
          tunnel: w318 -> [w328 w329 w330 w331 w332 w333 _ w343]
          frame "LINEA 135A BYPASS TRASFO", Default {
          }
          frame "LINEA 15A BYPASS TRASFO" {
          }
          frame "LINEA 135A TRASFO 400V" {
          }
          frame "LINEA 135A TRASFO 500V" {
          }
          frame "LINEA 15A TRASFO 400V" {
          }
          frame "LINEA 15A TRASFO 500V" {
          }
          frame "LINEA 2" {
            # "VACON"
            n157 = global read "STATUS VACON.vi" "STATUS VACON"() -> (w335:T38)
            n158 = Unbundle By Name(w335) -> ("RUN"=w334:bool)
            n159 = Obtain Queue(name (unnamed)="VACON" ("name"), element data type=cluster{"DATA":variant, "status":string} {"DATA"=variant, "status"=""} ("output cluster"), create if not found? (T)=TRUE) -> (queue out=w340:refnum<queue>)  [unwired: 2 in, 2 out]
            n160 = Bundle By Name(cluster=cluster{"DATA":variant, "status":string} {"DATA"=variant, "status"="Run command"} ("element"), "DATA"=TRUE) -> (w337:cluster{"DATA":variant, "status":string})
            n161 = Enqueue Element(queue=w340, element=w337) -> ()  [unwired: 2 in, 3 out]
          }
          frame "NESSUNA LINEA SELEZIONATA" {
          }
        }
        n162 = Select(t="Fine avvio", s=w320, f=w324) -> (s? t:f=w323:string)
      }
      frame "Fine avvio" {
        n163 = global write "Global_bypass_ResMeter.vi" "Bypass res meter"(FALSE ("Bypass res meter")) -> ()
      }
    }
  }
  "Fine Avvio" <- w8
  "Stato" <- w2
